vi "ConvTool.vi"() -> ()   [LabVIEW 2015]
panel:
  in  "取消按钮":bool
  in  "刷新按钮":bool
  in  "DEC":string
  in  "String":string
  in  "HEX":string
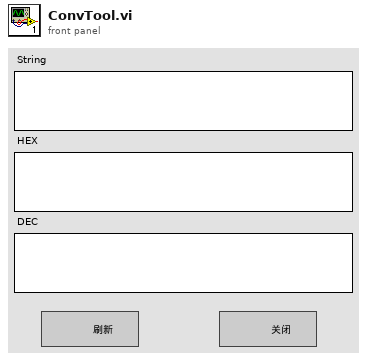
[diagram p1: front panel]
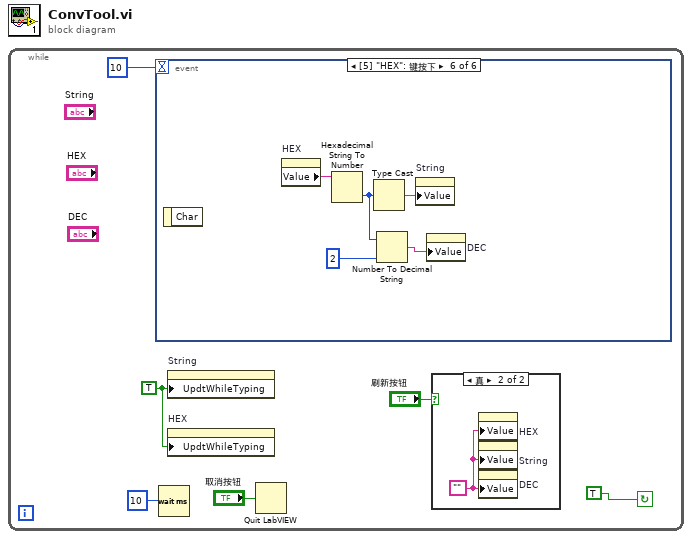
[diagram p0: block diagram]
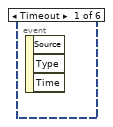
[diagram p3: hidden frame]
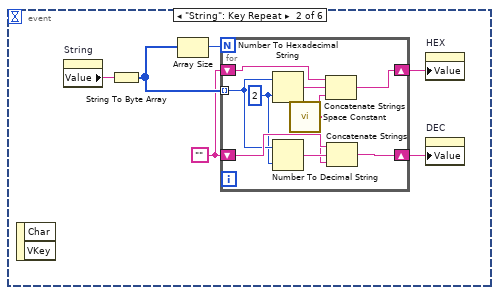
[diagram p4: hidden frame]
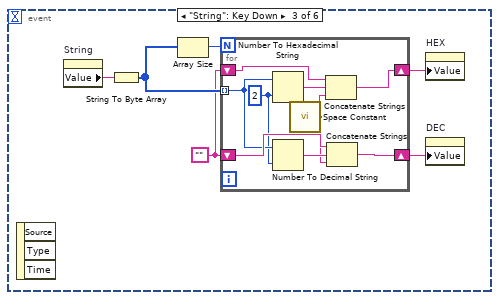
[diagram p5: hidden frame]
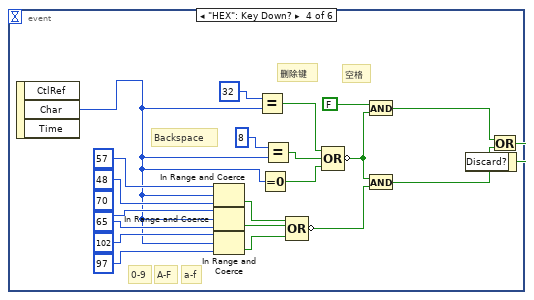
[diagram p6: hidden frame]
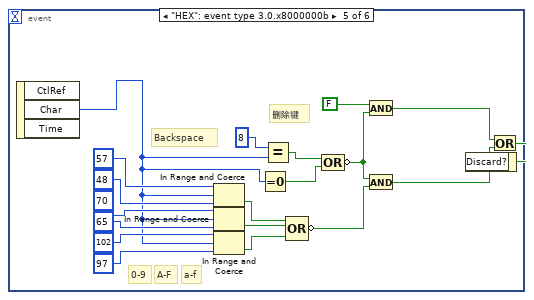
[diagram p7: hidden frame]
diagram:
  n1 = while {
    stop <- TRUE continue-if-true
    w3 = TRUE
    n2 = event shown="[5] \"HEX\": 键按下" {
      selector: _ -> [_ _ _ _ _ _]
      dyn-events: _ -> [_ _ _ _ _ _]
      timeout: 10 -> [_ _ _ _ _ _]
      event Timeout {
        n3 = event-data() -> ()  [unwired: 1 in, 3 out]
      }
      event "String": Key Repeat {
        w9 = ""
        n4 = event-data() -> ()  [unwired: 1 in, 2 out]
        n5 = property on="String" class="Str"() -> ("Value"=w13:string)  [unwired: 2 in, 2 out]
        n6 = String To Byte Array(string=w13) -> (unsigned byte array=w11:u8[])
        n7 = Array Size(array=w11) -> (size(s)=w10:i32)
        n8 = for {
          N: w10 -> [_]
          tunnel: w11 -> [w18] mode=indexing
          shift-right: [w21] -> w12
          shift-left: w9 -> [w20]
          shift-right: [w15] -> w8
          shift-left: w9 -> [w14]
          w17 = 2
          n9 = Number To Hexadecimal String(1:w17, 2:w18) -> (0:w16:string)
          n10 = Number To Decimal String(number=w18, width (-)=w17) -> (decimal integer string=w22:string)
          n11 = call <vilib>:"Space Constant.vi"() -> ("String"=w19:string)
          n12 = Concatenate Strings(w14, w16, w19) -> (w15:string)
          n13 = Concatenate Strings(w20, w22, w19) -> (w21:string)
        }
        n14 = property on="HEX" class="Str"("Value"=w8) -> ()  [unwired: 2 in, 2 out]
        n15 = property on="DEC" class="Str"("Value"=w12) -> ()  [unwired: 2 in, 2 out]
      }
      event "String": Key Down {
        w24 = ""
        n16 = event-data() -> ()  [unwired: 1 in, 3 out]
        n17 = property on="String" class="Str"() -> ("Value"=w28:string)  [unwired: 2 in, 2 out]
        n18 = String To Byte Array(string=w28) -> (unsigned byte array=w26:u8[])
        n19 = Array Size(array=w26) -> (size(s)=w25:i32)
        n20 = for {
          N: w25 -> [_]
          tunnel: w26 -> [w33] mode=indexing
          shift-right: [w36] -> w27
          shift-left: w24 -> [w35]
          shift-right: [w30] -> w23
          shift-left: w24 -> [w29]
          w32 = 2
          n21 = Number To Hexadecimal String(1:w32, 2:w33) -> (0:w31:string)
          n22 = Number To Decimal String(number=w33, width (-)=w32) -> (decimal integer string=w37:string)
          n23 = call <vilib>:"Space Constant.vi"() -> ("String"=w34:string)
          n24 = Concatenate Strings(w29, w31, w34) -> (w30:string)
          n25 = Concatenate Strings(w35, w37, w34) -> (w36:string)
        }
        n26 = property on="HEX" class="Str"("Value"=w23) -> ()  [unwired: 2 in, 2 out]
        n27 = property on="DEC" class="Str"("Value"=w27) -> ()  [unwired: 2 in, 2 out]
      }
      event "HEX": Key Down? {
        # "空格"
        # "删除键"
        # "a-f"
        # "A-F"
        # "0-9"
        # "Backspace"
        n28 = event-data() -> ("Char"=w40:i16)  [unwired: 1 in, 2 out]
        n29 = In Range and Coerce(upper limit=i16 57, x=w40, lower limit=i16 48) -> (In Range?=w47:bool)  [unwired: 1 out]
        n30 = In Range and Coerce(upper limit=i16 70, x=w40, lower limit=i16 65) -> (In Range?=w48:bool)  [unwired: 1 out]
        n31 = In Range and Coerce(upper limit=i16 102, x=w40, lower limit=i16 97) -> (In Range?=w55:bool)  [unwired: 1 out]
        n32 = Equal?(x=i16 32, y=w40) -> (x = y?=w38:bool)
        n33 = Equal To 0?(x=w40) -> (x = 0?=w57:bool)
        n34 = Equal?(x=i16 8, y=w40) -> (x = y?=w56:bool)
        n35 = Compound Arithmetic op=OR ("复合运算")(w47, w48, w55) -> (invert w53:bool)
        n36 = Compound Arithmetic op=OR ("复合运算")(w38, w56, w57) -> (invert w58:bool)
        n37 = And(x=FALSE, y=w58) -> (x .and. y?=w52:bool)
        n38 = And(x=w58, y=w53) -> (x .and. y?=w54:bool)
        n39 = Or(x=w52, y=w54) -> (x .or. y?=w42:bool)
        n40 = event-data("Discard?"=w42) -> ()  [unwired: 1 in, 1 out]
      }
      event "HEX": event type 3.0.x8000000b {
        # "删除键"
        # "a-f"
        # "A-F"
        # "0-9"
        # "Backspace"
        n41 = event-data() -> ("Char"=w61:i16)  [unwired: 1 in, 2 out]
        n42 = In Range and Coerce(upper limit=i16 57, x=w61, lower limit=i16 48) -> (In Range?=w66:bool)  [unwired: 1 out]
        n43 = In Range and Coerce(upper limit=i16 70, x=w61, lower limit=i16 65) -> (In Range?=w67:bool)  [unwired: 1 out]
        n44 = In Range and Coerce(upper limit=i16 102, x=w61, lower limit=i16 97) -> (In Range?=w74:bool)  [unwired: 1 out]
        n45 = Equal To 0?(x=w61) -> (x = 0?=w76:bool)
        n46 = Equal?(x=i16 8, y=w61) -> (x = y?=w75:bool)
        n47 = Compound Arithmetic op=OR ("复合运算")(w66, w67, w74) -> (invert w72:bool)
        n48 = Compound Arithmetic op=OR ("复合运算")(w75, w76) -> (invert w77:bool)
        n49 = And(x=FALSE, y=w77) -> (x .and. y?=w71:bool)
        n50 = And(x=w77, y=w72) -> (x .and. y?=w73:bool)
        n51 = Or(x=w71, y=w73) -> (x .or. y?=w60:bool)
        n52 = event-data("Discard?"=w60) -> ()  [unwired: 1 in, 1 out]
      }
      event "HEX": Key Down {
        n53 = event-data() -> ()  [unwired: 1 in, 1 out]
        n54 = property on="HEX" class="Str"() -> ("Value"=w82:string)  [unwired: 2 in, 2 out]
        n55 = Hexadecimal String To Number(string=w82) -> (number=w80:u32)  [unwired: 2 in, 1 out]
        n56 = Type Cast(x=w80) -> (*(type *) &x=w81:string)  [unwired: 1 in]
        n57 = Number To Decimal String(number=w80, width (-)=2) -> (decimal integer string=w79:string)
        n58 = property on="String" class="Str"("Value"=w81) -> ()  [unwired: 2 in, 2 out]
        n59 = property on="DEC" class="Str"("Value"=w79) -> ()  [unwired: 2 in, 2 out]
      }
    }
    n60 = Wait (ms)(milliseconds to wait=10) -> ()  [unwired: 1 out]
    n61 = property on="String" class="Str"("UpdtWhileTyping"=w3) -> ()  [unwired: 2 in, 2 out]
    n62 = property on="HEX" class="Str"("UpdtWhileTyping"=w3) -> ()  [unwired: 2 in, 2 out]
    n63 = Quit LabVIEW(quit? (T)="取消按钮") -> ()
    n64 = case shown="真" "刷新按钮" {
      frame False {
      }
      frame True {
        w7 = ""
        n65 = property on="HEX" class="Str"("Value"=w7) -> ()  [unwired: 2 in, 2 out]
        n66 = property on="String" class="Str"("Value"=w7) -> ()  [unwired: 2 in, 2 out]
        n67 = property on="DEC" class="Str"("Value"=w7) -> ()  [unwired: 2 in, 2 out]
      }
    }
  }
